vi "Create.vi"(0 "Name":string, 1 "ID":i32=-1, 5 "Path":string, 7 "Type":T1, 9 "Parent ID":i32=-1, 11 "error in (no error)":errorcluster) -> (4 "Object out":refnum<class "Object.lvclass">, 15 "error out":errorcluster)   [LabVIEW 2019, in "HierDAL Library.lvlib" / "Models.lvlib" / "Object.lvclass"]
uses:
  Object.lvclass
  Controls/Datatype.ctl
  Attribute Class/Attribute.lvclass
  Object.lvclass/Object.ctl
  HierDAL Library.lvlib
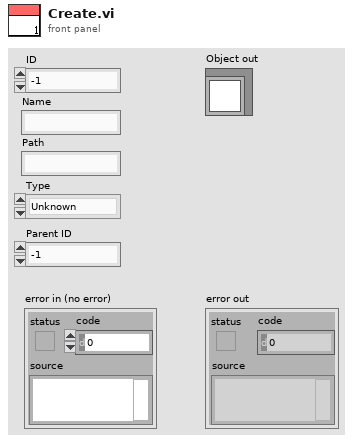
[diagram p1: front panel]
types:
  T1 = typedef "HierDAL Library.lvlib/Datatype.ctl" = enum16{"Unknown", "Group", "Dataset"}
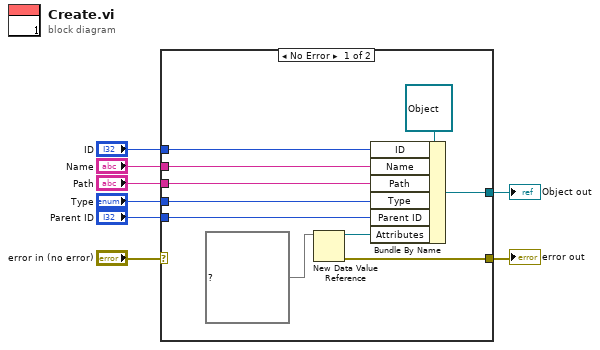
[diagram p0: block diagram]
diagram:
  n1 = case shown="No Error" "error in (no error)" {
    selector: "error in (no error)" -> [_ w19]
    tunnel: [w17 _] -> w8
    tunnel: [w15 w19] -> w7
    tunnel: "ID" -> [w13 _]
    tunnel: "Name" -> [w12 _]
    tunnel: "Path" -> [w11 _]
    tunnel: "Type" -> [w10 _]
    tunnel: "Parent ID" -> [w9 _]
    frame No Error {
      n2 = New Data Value Reference(data value=map{string, refnum<class "Attribute.lvclass">} {} ("map")) -> (data value reference=w14:refnum<data-value>, error out=w15:errorcluster)  [unwired: 1 in]
      n3 = Bundle By Name(cluster=refnum<class "Object.lvclass"> refnum ("Object out"), "ID"=w13, "Name"=w12, "Path"=w11, "Type"=w10, "Parent ID"=w9, "Attributes"=w14) -> (w17:refnum<class "Object.lvclass">)
    }
    frame Error {
    }
  }
  "error out" <- w7
  "Object out" <- w8
